vi "Draw ROI.vi"(8 "error in (no error)":errorcluster, 9 "结果":bool, 10 "Rectangle":T2 {"Rotation" format="%.2f"; "Left" scale=0.0..1024.0; "Right" scale=0.0..1024.0}, 11 "处理后图像 In":T1(plugin-control)) -> (0 "error out":errorcluster, 3 "处理后图像 Out":T1(plugin-control))   [LabVIEW 2017]
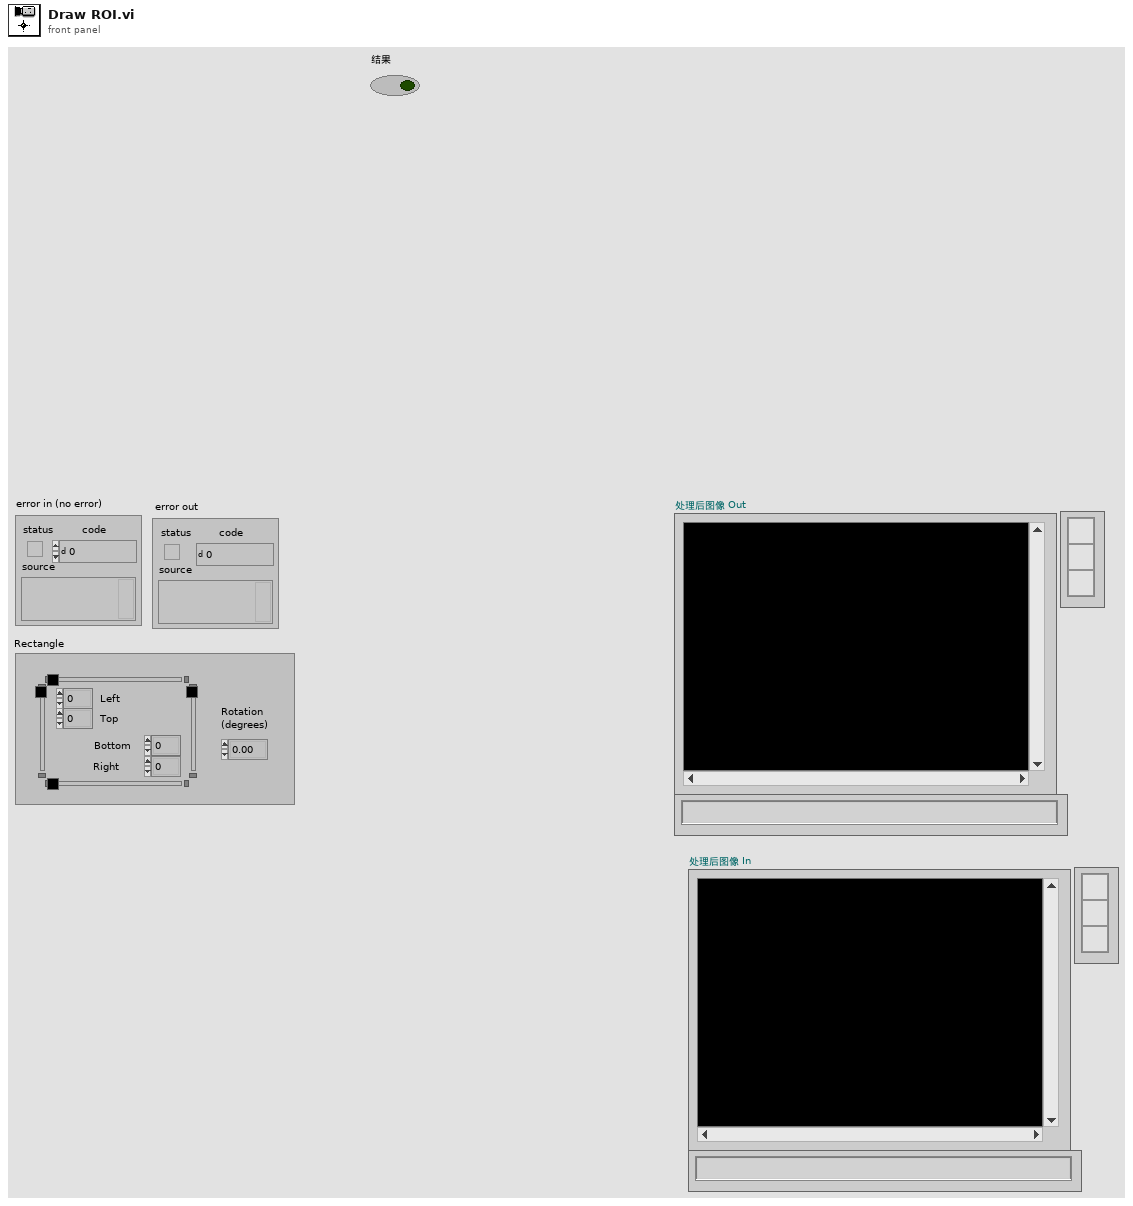
[diagram p1: front panel]
types:
  T1 = typedef "IMAQ Image.ctl" = refnum<image>
  T2 = typedef "IMAQ Rectangle" = cluster{"Left":i32, "Top":i32, "Right":i32, "Bottom":i32, "Rotation":dbl}
  T3 = cluster{"Desired Font (Application)":enum16{"User-specified Font", "Application Font", "System Font", "Dialog Font"}, "[User-specified Font]":cluster{"Font Name":string, "Size":i16, "Strikeout?":bool, "Italic?":bool, "Underline?":bool, "Outline?":bool, "Shadow?":bool, "Bold?":bool, "Rotation Angle":dbl}, "Horizontal Alignment":i16, "Vertical Alignment":i16}
  T4 = cluster{"Left":i32, "Top":i32, "Right":i32, "Bottom":i32}
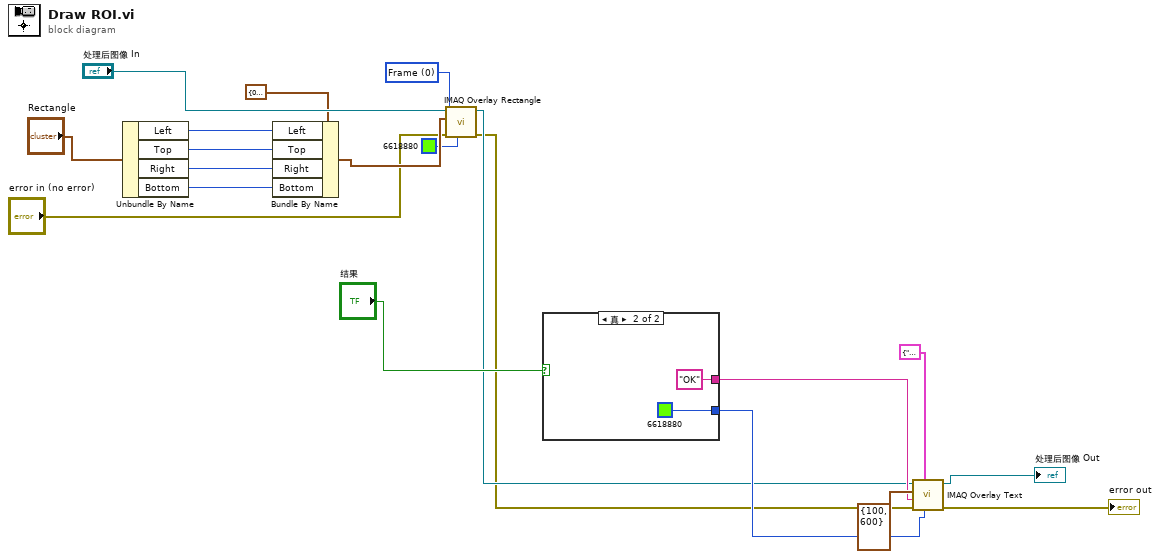
[diagram p0: block diagram]
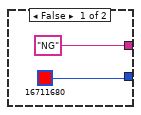
[diagram p2: hidden frame]
diagram:
  w11 = u32 0 items=["Frame", "Fill", "Highlight"] ("Drawing Mode (Frame)")
  n1 = Unbundle By Name("Rectangle") -> ("Left"=w17:i32, "Top"=w16:i32, "Right"=w15:i32, "Bottom"=w14:i32)
  n2 = Bundle By Name(cluster=T4 {"Left"=0, "Top"=0, "Right"=0, "Bottom"=0} ("Rectangle"), "Left"=w17, "Top"=w16, "Right"=w15, "Bottom"=w14) -> (w13:T4)
  n3 = call "IMAQ Overlay Rectangle"("Color"=u32 6618880, "error in (no error)"="error in (no error)", "Drawing Mode (Frame)"=w11, "Rectangle"=w13, "Image"="处理后图像 In") -> ("error out"=w3:errorcluster, "Image Out"=w4:T1)  [unwired: 5 in]
  n4 = case shown="真" "结果" {
    tunnel: ["NG" "OK"] -> w7
    tunnel: [u32 16711680 ("Text Color (black)") u32 6618880 ("Text Color (black)")] -> w5
    frame False {
    }
    frame True {
    }
  }
  n5 = call "IMAQ Overlay Text"("Text Color (black)"=w5, "Font, Size & Style"=T3 {"Desired Font (Application)"=enum."User-specified Font", "[User-specified Font]"={"Font Name"="", "Size"=400, "Strikeout?"=FALSE, "Italic?"=FALSE, "Underline?"=FALSE, "Outline?"=FALSE, "Shadow?"=FALSE, "Bold?"=TRUE, "Rotation Angle"=0.0}, "Horizontal Alignment"=0, "Vertical Alignment"=0}, "error in (no error)"=w3, "String"=w7, "Origin"=cluster{"X":i32, "Y":i32} {"X"=100, "Y"=600}, "Image"=w4) -> ("error out"=→"error out":errorcluster, "Image Out"=→"处理后图像 Out":T1)  [unwired: 4 in]
